vi "ActivateHW.vi"(8 "error in (no error)":errorcluster, 11 "BME_DG_Base in":refnum<class "BME_DG_Base.lvclass">) -> (0 "error out":errorcluster, 3 "BME_DG_Base out":refnum<class "BME_DG_Base.lvclass">)   [LabVIEW 2009, in "POLARIS BME DG.lvlib" / "BME_DG_Base.lvclass"]
uses:
  BME_DG_Base.lvclass
  BME_DG_Base.lvclass/BME_DG_Base.ctl
  POLARIS BME DG.lvlib
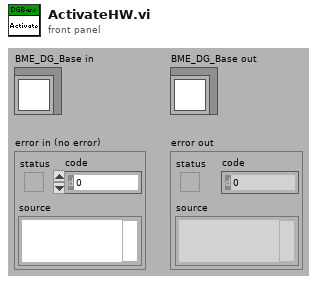
[diagram p1: front panel]
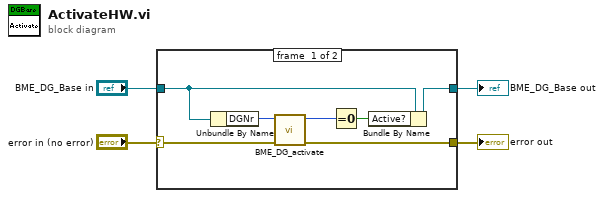
[diagram p0: block diagram]
diagram:
  n1 = case shown="No Error" "error in (no error)" {
    selector: "error in (no error)" -> [w11 w13]
    tunnel: [w10 w13] -> w3
    tunnel: [w7 w12] -> w1
    tunnel: "BME_DG_Base in" -> [w9 w12]
    frame #0 {
      n2 = Unbundle By Name(w9) -> ("DGNr"=w8:i32)
      n3 = call "BME_DG_activate.vi"("error in (no error)"=w11, "DG_Number"=w8) -> ("error out"=w10:errorcluster, "return code"=w6:i32)  [unwired: 8 in]
      n4 = Equal To 0?(x=w6) -> (x = 0?=w5:bool)
      n5 = Bundle By Name(cluster=w9, "Active?"=w5) -> (w7:refnum<class "BME_DG_Base.lvclass">)
    }
    frame #1 {
    }
  }
  "error out" <- w3
  "BME_DG_Base out" <- w1
